vi "gain setting to gain.vi"(10 "Gain setting":u8) -> (2 "gain":dbl)   [LabVIEW 2017]
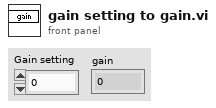
[diagram p1: front panel]
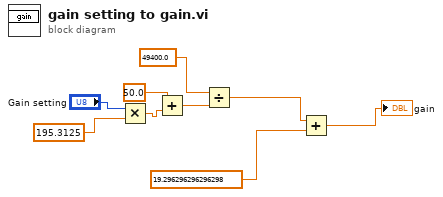
[diagram p0: block diagram]
diagram:
  n1 = Multiply(x="Gain setting", y=195.3125) -> (x*y=w7:dbl)
  n2 = Add(x=50.0, y=w7) -> (x+y=w5:dbl)
  n3 = Divide(x=49400.0, y=w5) -> (x/y=w3:dbl)
  n4 = Add(x=w3, y=19.296296296296298) -> (x+y=→"gain":dbl)
